vi "jsq_decode.vi"(8 "error in":errorcluster, 10 "JSON string":string="[\r\n]") -> (0 "error out":errorcluster, 2 "Sequence":T1[](array[typedef]))   [LabVIEW 2015, in "oskar_tools.lvlib"]
uses:
  oskar_tools.lvlib
  seq_line.ctl
  <vilib>/regexp/Match Regular Expression.xnode
  <vilib>/addons/_JKI.lib/Serialization/JSON/JKI JSON Serialization.lvlib
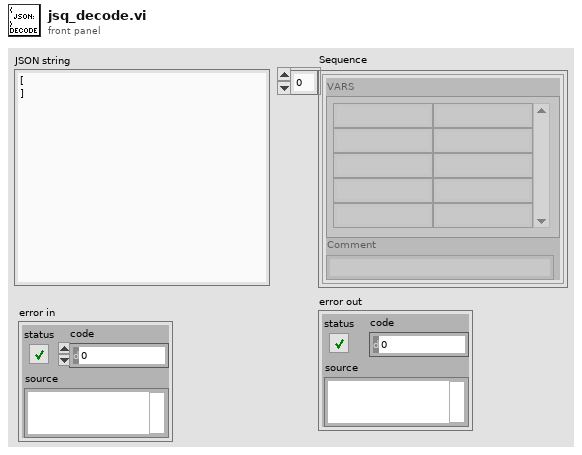
[diagram p1: front panel]
types:
  T1 = typedef "oskar_tools.lvlib/seq_line.ctl" = cluster{"VARS":string[][], "Comment":string}
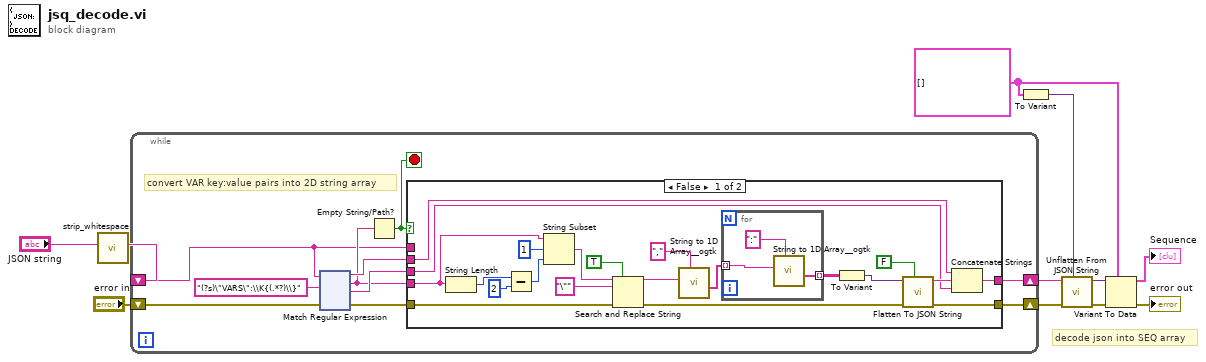
[diagram p0: block diagram]
diagram:
  w7 = T1[] [] ("Sequence 2")
  # "decode json into SEQ array"
  n1 = call "strip_whitespace.vi"("String in"="JSON string") -> ("String out"=w10:string)  [unwired: 10 in]
  n2 = while {
    shift-right: [w18] -> w9
    shift-left: w10 -> [w16]
    shift-right: [w12] -> w3
    shift-left: "error in" -> [w14]
    stop <- w15 stop-if-true
    # "convert VAR key:value pairs into 2D string array"
    n3 = xnode "Match Regular Expression"("input string"=w16, "regular expression"="(?s)\"VARS\":\\K{(.*?)\\}", "error in"=w14) -> ("before match"=w20:string, "whole match"=w17:string, "after match"=w19:string, "error out"=w13:errorcluster)  [unwired: 3 in, 1 out]
    n4 = Empty String/Path?(string/path=w17) -> (empty?=w15:bool)
    n5 = case shown="False" w15 {
      tunnel: w20 -> [w31 _]
      tunnel: w19 -> [w29 _]
      tunnel: [w28 w47] -> w18
      tunnel: w17 -> [w25 _]
      tunnel: w16 -> [_ w47]
      tunnel: w13 -> [w24 w46]
      tunnel: [w22 w46] -> w12
      frame False {
        n6 = String Length(string=w25) -> (length=w41:i32)
        n7 = Subtract(x=w41, y=2) -> (x-y=w39:i32)
        n8 = String Subset(string=w25, offset (0)=1, length (rest)=w39) -> (substring=w37:string)
        n9 = Search and Replace String(replace all?=TRUE ("replace all? (F)"), input string=w37, search string="\"", error in=w24) -> (result string=w34:string, error out=w23:errorcluster)  [unwired: 4 in, 2 out]
        n10 = call <userlib>:"String to 1D Array__ogtk.vi"("delimiter (Tab)"=",", "string"=w34) -> ("Array of Strings"=w33:string[])  [unwired: 9 in]
        n11 = for {
          tunnel: w33 -> [w45] mode=indexing
          tunnel: [w43] -> w27 mode=indexing
          n12 = call <userlib>:"String to 1D Array__ogtk.vi"("delimiter (Tab)"=":", "string"=w45) -> ("Array of Strings"=w43:string[])  [unwired: 9 in]
        }
        n13 = To Variant(anything=w27) -> (Variant=w26:variant)
        n14 = call <vilib>:"Flatten To JSON String.vi"("Multiline (T)"=FALSE, "error in (no error)"=w23, "Variant"=w26) -> ("error out"=w22:errorcluster, "JSON String"=w30:string)  [unwired: 7 in]
        n15 = Concatenate Strings(w31, w30, w29) -> (w28:string)
      }
      frame True {
      }
    }
  }
  n16 = To Variant(anything=w7) -> (Variant=w8:variant)
  n17 = call <vilib>:"Unflatten From JSON String.vi"("Type and Defaults"=w8, "error in (no error)"=w3, "JSON String"=w9) -> ("error out"=w2:errorcluster, "Variant"=w6:variant)  [unwired: 7 in]
  n18 = Variant To Data(error in=w2, type=w7, Variant=w6) -> (data=→"Sequence":T1[], error out=→"error out":errorcluster)
